vi "GroveFirmwareVersionCheck.vi"() -> ()   [LabVIEW 2014]
doc: "GrovePi example for checking the firmware version of the GrovePi."
uses:
  <vilib>/MakerHub/LINX/Public/Utilities/Open Local.vi
  LinxGrovePi/LinxGrovePi.lvclass
  <vilib>/MakerHub/LINX/LMH-LINX.lvlib
panel:
  out "Firmware Version":string
  out "Error Out":errorcluster
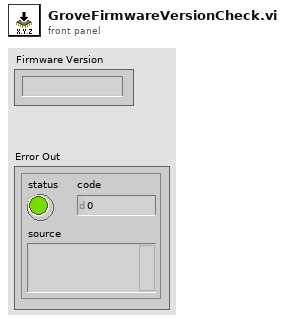
[diagram p1: front panel]
types:
  T1 = typedef "LMH-LINX.lvlib/LINX Ref.ctl" = cluster{"IO":T2, "Interface":T3, "LINX Device Config":T4}
  T2 = typedef "LMH-LINX.lvlib/Platform.ctl" = enum16{"Remote", "Local"}
  T3 = typedef "LMH-LINX.lvlib/Interface.ctl" = enum16{"Serial", "TCP"}
  T4 = typedef "LMH-LINX.lvlib/Device.lvlib/LINX Device Config.ctl" = cluster{"Interface":T3, "COM Port":refnum<visa-resource-name>, "TCP Configuration":T5, "Device Family":u8, "Device ID":u8, "Device Name":string, "TCP Ref":refnum<k5>, "Channels":T6}
  T5 = typedef "LMH-LINX.lvlib/Device.lvlib/TCP Config.ctl" = cluster{"IP Address":string, "Port":u16}
  T6 = typedef "LMH-LINX.lvlib/Channels.ctl" = cluster{"DI":u8[], "DO":u8[], "AI":u8[], "AO":u8[], "PWM":u8[], "QE":u8[], "UART":u8[], "I2C 2":u8[], "SPI":u8[], "CAN":u8[], "Servo":u8[], "AI Ref (V)":dbl, "AI Resolution (Bits)":u8, "AO Ref (V)":dbl, "AO Resolution (Bits)":u8}
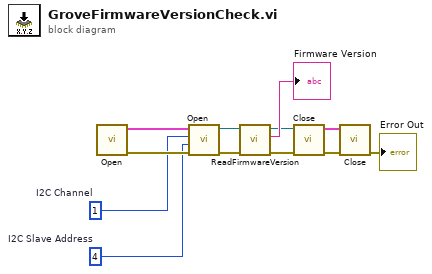
[diagram p0: block diagram]
diagram:
  w8 = u8 4  # I2C Slave Address
  w9 = u8 1  # I2C Channel
  n1 = call-poly <vilib>:"Open.vi"() -> ("Error Out"=w10:errorcluster, "LINX Resource"=w11:T1)  [unwired: 9 in, 1 out]
  n2 = call <vilib>:"Open.vi"("error in (no error)"=w10, "I2C Slave Address (4)"=w8, "I2C Channel (1)"=w9, "LINX Resource"=w11) -> ("error out"=w5:errorcluster, "LINX GrovePi out"=w4:refnum<class "LinxGrovePi.lvclass">)  [unwired: 6 in]
  n3 = call-dynamic "ReadFirmwareVersion.vi"("error in (no error)"=w5, "GrovePi in"=w4) -> ("error out"=w1:errorcluster, "Firmware Version"=→"Firmware Version":string, "GrovePi out"=w2:refnum<class "LinxGrovePi.lvclass">)  [unwired: 7 in]
  n4 = call <vilib>:"Close.vi"("error in (no error)"=w1, "LINX GrovePi in"=w2) -> ("error out"=w6:errorcluster, "LINX Resource"=w7:T1)  [unwired: 8 in]
  n5 = call <vilib>:"Close.vi"("Error In"=w6, "LINX Resource"=w7) -> ("Error Out"=→"Error Out":errorcluster)  [unwired: 9 in]
